vi "Simon.vi"() -> ()   [LabVIEW 2025]
panel:
  out "Array Size":dbl
  out "Current State":string
  in  "start":bool
  in  "stop":bool
  out "Blue":bool
  out "Yellow":bool
  out "Red":bool
  out "Green":bool
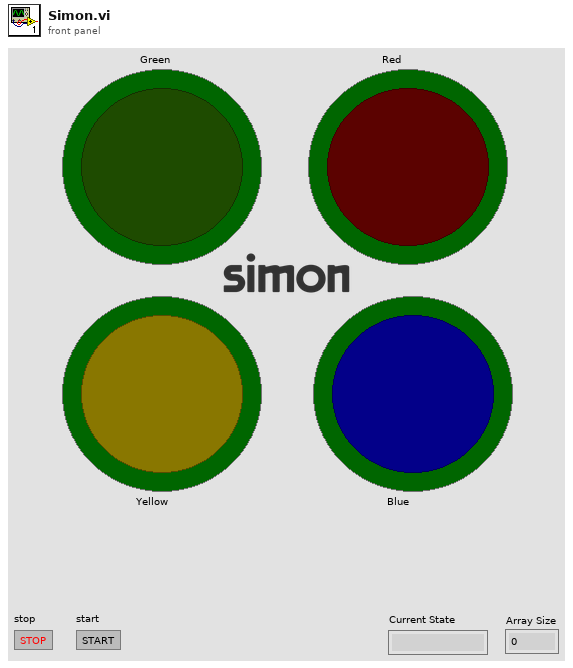
[diagram p1: front panel]
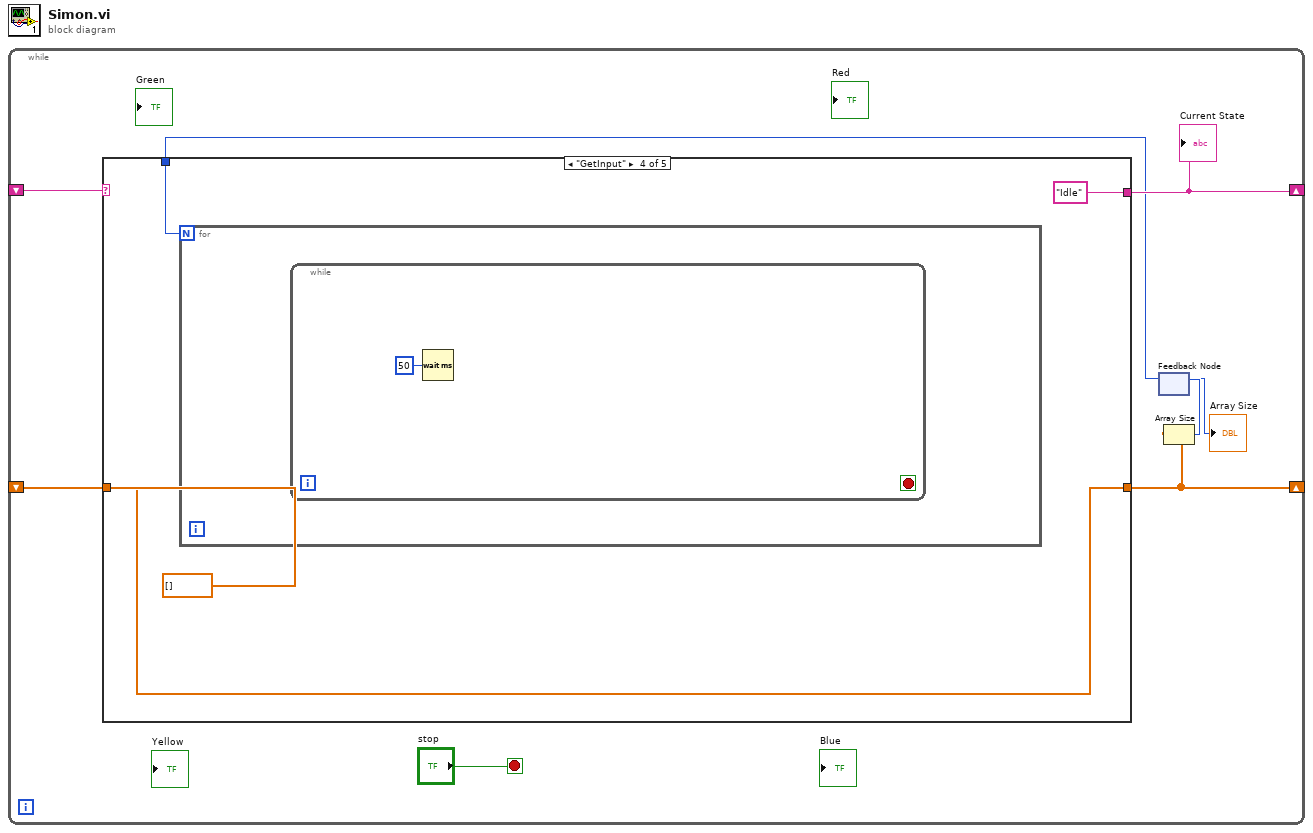
[diagram p0: block diagram]
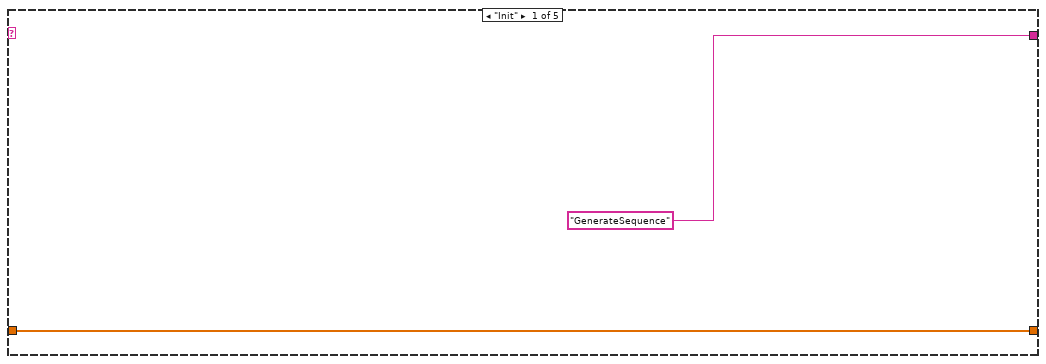
[diagram p2: hidden frame]
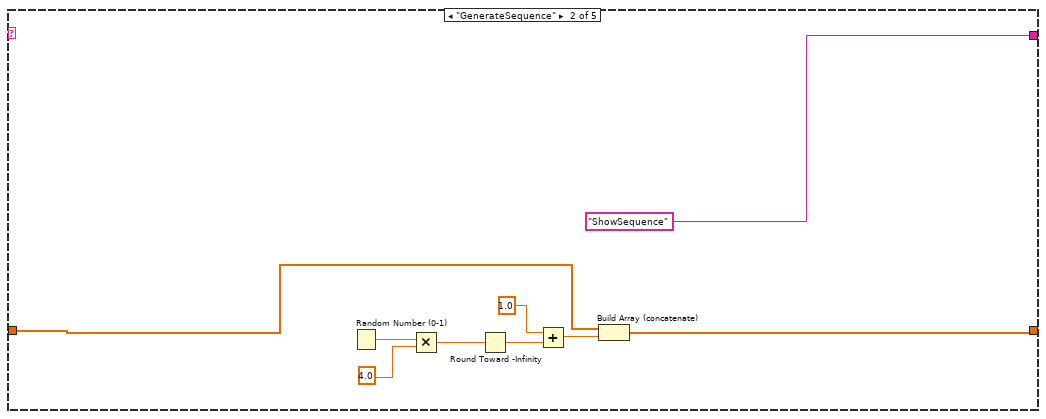
[diagram p3: hidden frame]
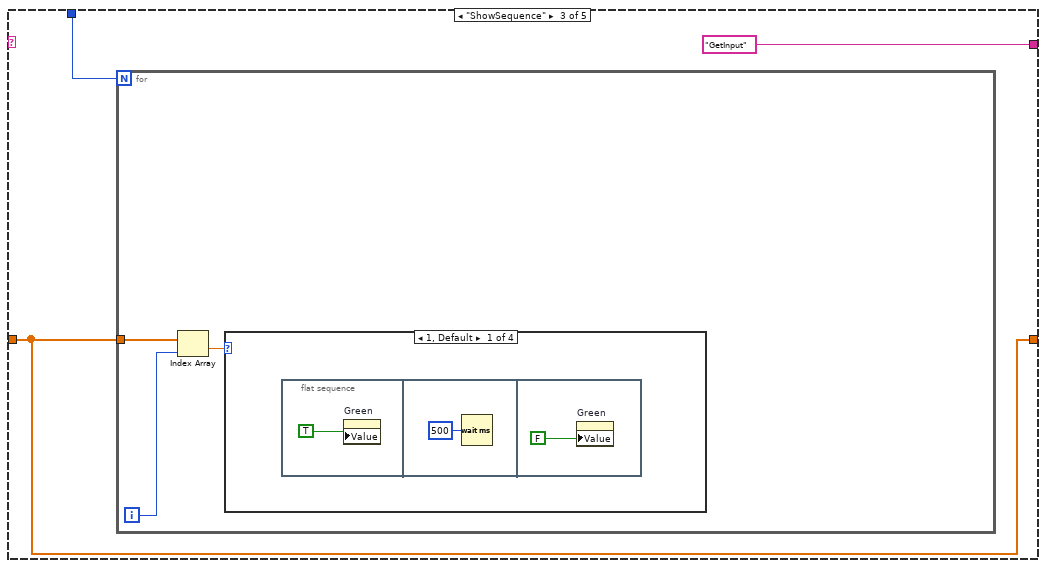
[diagram p4: hidden frame]
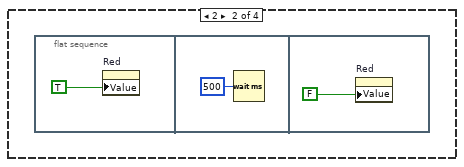
[diagram p5: hidden frame]
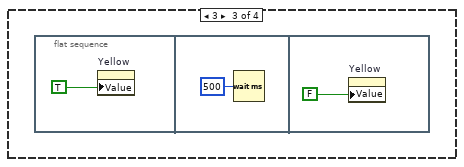
[diagram p6: hidden frame]
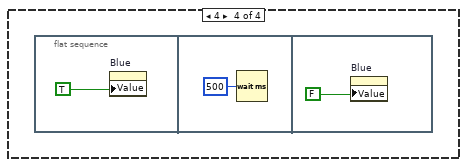
[diagram p7: hidden frame]
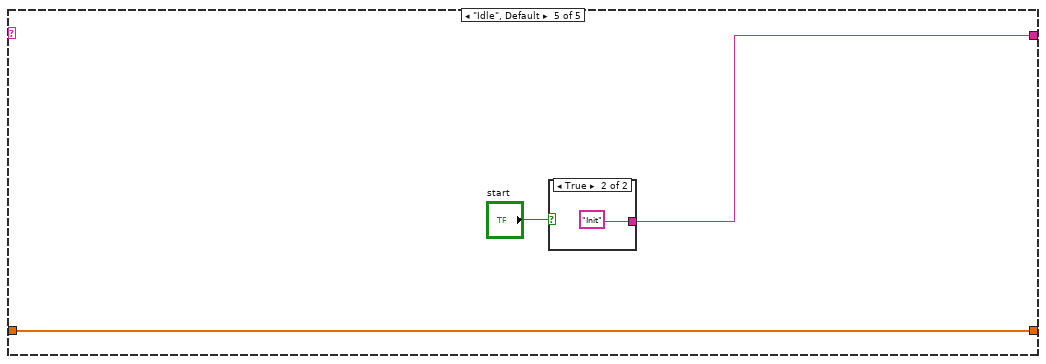
[diagram p8: hidden frame]
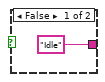
[diagram p9: hidden frame]
diagram:
  n1 = while {
    shift-right: [w7] -> _
    shift-left: _ -> [w5]
    shift-right: [w4] -> _
    shift-left: dbl[] [] -> [w6]
    stop <- "stop" stop-if-true
    n2 = feedback #1() -> (w2:i32)  [unwired: 1 in]
    "Array Size" <- w2
    n3 = case shown="\"GetInput\"" w5 {
      tunnel: ["GenerateSequence" "ShowSequence" "GetInput" "Idle" w43] -> w7
      tunnel: [w9 w12 w20 w39 w42] -> w4
      tunnel: w6 -> [w9 w13 w20 w39 w42]
      tunnel: w2 -> [_ _ w21 w38 _]
      frame "Init" {
      }
      frame "GenerateSequence" {
        n4 = Random Number (0-1)() -> (number: 0 to 1=w19:dbl)
        n5 = Multiply(x=w19, y=4.0) -> (x*y=w17:dbl)
        n6 = Round Toward -Infinity(1:w17) -> (0:w15:dbl)
        n7 = Add(x=1.0, y=w15) -> (x+y=w14:dbl)
        n8 = Build Array (concatenate)(w13, w14) -> (w12:dbl[])
      }
      frame "ShowSequence" {
        n9 = for {
          N: w21 -> [_]
          tunnel: w20 -> [w25]
          i -> [w24]
          n10 = Index Array(array=w25, index=w24) -> (element=w23:dbl)
          n11 = case shown="1, Default" w23 {
            frame 1, Default {
              n12 = flat-sequence {
                frame #0 {
                  n13 = property on="Green" class="Bool (strict)"("Value"=TRUE) -> ()  [unwired: 2 in, 2 out]
                }
                frame #1 {
                  n14 = Wait (ms)(milliseconds to wait=u32 500) -> ()  [unwired: 1 out]
                }
                frame #2 {
                  n15 = property on="Green" class="Bool (strict)"("Value"=FALSE) -> ()  [unwired: 2 in, 2 out]
                }
              }
            }
            frame 2 {
              n16 = flat-sequence {
                frame #0 {
                  n17 = property on="Red" class="Bool (strict)"("Value"=TRUE) -> ()  [unwired: 2 in, 2 out]
                }
                frame #1 {
                  n18 = Wait (ms)(milliseconds to wait=u32 500) -> ()  [unwired: 1 out]
                }
                frame #2 {
                  n19 = property on="Red" class="Bool (strict)"("Value"=FALSE) -> ()  [unwired: 2 in, 2 out]
                }
              }
            }
            frame 3 {
              n20 = flat-sequence {
                frame #0 {
                  n21 = property on="Yellow" class="Bool (strict)"("Value"=TRUE) -> ()  [unwired: 2 in, 2 out]
                }
                frame #1 {
                  n22 = Wait (ms)(milliseconds to wait=u32 500) -> ()  [unwired: 1 out]
                }
                frame #2 {
                  n23 = property on="Yellow" class="Bool (strict)"("Value"=FALSE) -> ()  [unwired: 2 in, 2 out]
                }
              }
            }
            frame 4 {
              n24 = flat-sequence {
                frame #0 {
                  n25 = property on="Blue" class="Bool (strict)"("Value"=TRUE) -> ()  [unwired: 2 in, 2 out]
                }
                frame #1 {
                  n26 = Wait (ms)(milliseconds to wait=u32 500) -> ()  [unwired: 1 out]
                }
                frame #2 {
                  n27 = property on="Blue" class="Bool (strict)"("Value"=FALSE) -> ()  [unwired: 2 in, 2 out]
                }
              }
            }
          }
        }
      }
      frame "GetInput" {
        n28 = for {
          N: w38 -> [_]
          n29 = while {
            stop <- _ stop-if-true
            n30 = Wait (ms)(milliseconds to wait=u32 50) -> ()  [unwired: 1 out]
          }
        }
      }
      frame "Idle", Default {
        n31 = case shown="True" "start" {
          tunnel: ["Idle" "Init"] -> w43
          frame False {
          }
          frame True {
          }
        }
      }
    }
    "Current State" <- w7
    n32 = Array Size(array=w4) -> (size(s)=w3:i32)
    n33 = feedback-in #1(w3) -> ()
  }
